vi "write acquisition config.vi"(8 "error in (no error)":errorcluster, 11 "Channel in":refnum<class "SPARC4_Channel.lvclass">) -> (0 "error out":errorcluster, 3 "Channel out":refnum<class "SPARC4_Channel.lvclass">)   [LabVIEW 2018, in "SPARC4_Channel.lvclass"]
uses:
  SPARC4_Channel.lvclass
  C:/Users/Denis/Desktop/S4ACS/S4ACS/Channel/Channel.lvclass
  SPARC4_Channel.lvclass/SPARC4_Channel.ctl
  Sim_CCD/Sim_CCD.lvclass
  Channel/Channel.lvclass
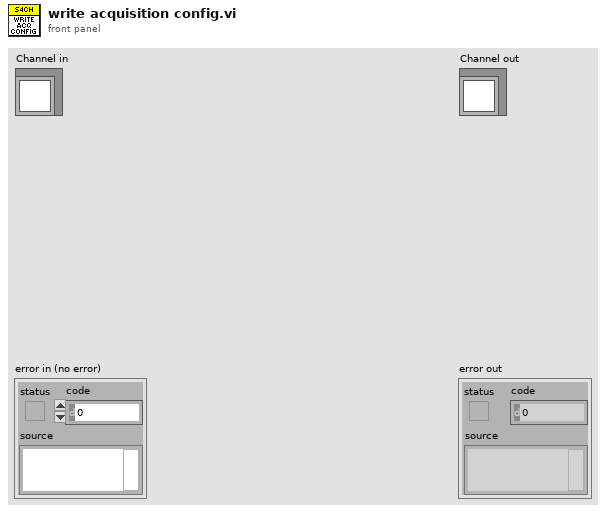
[diagram p1: front panel]
types:
  T1 = cluster{"#CYCLES":errorcluster, "SUFFIX":errorcluster}
  T2 = cluster{"#SEQS":errorcluster, "WAVEPLATE_POS":errorcluster}
  T3 = cluster{"State Machine.lvclass":refnum<class "State Machine.lvclass">, "RxTx.lvclass":refnum<class "RxTx.lvclass">, "Save_Header_RxTx.lvclass":refnum<class "RxTx.lvclass">, "Status SM.lvclass":refnum<class "State Machine.lvclass">, "Status RxTx.lvclass":refnum<class "RxTx.lvclass">, "servers array":refnum<class "Server.lvclass">[], "Events log file.lvclass":refnum<class "Log File.lvclass">, "Errors log file.lvclass":refnum<class "Log File.lvclass">, "Keywords log file.lvclass":refnum<class "Log File.lvclass">, "Sim_CCD.lvclass":refnum<class "Sim_CCD.lvclass">}
  T4 = cluster{"EXPTIME":errorcluster, "#FRAMES":errorcluster}
  T5 = cluster{"#SEQS":u32, "WAVEPLATE_POS":u16, "Waveplate positions":u8[]}
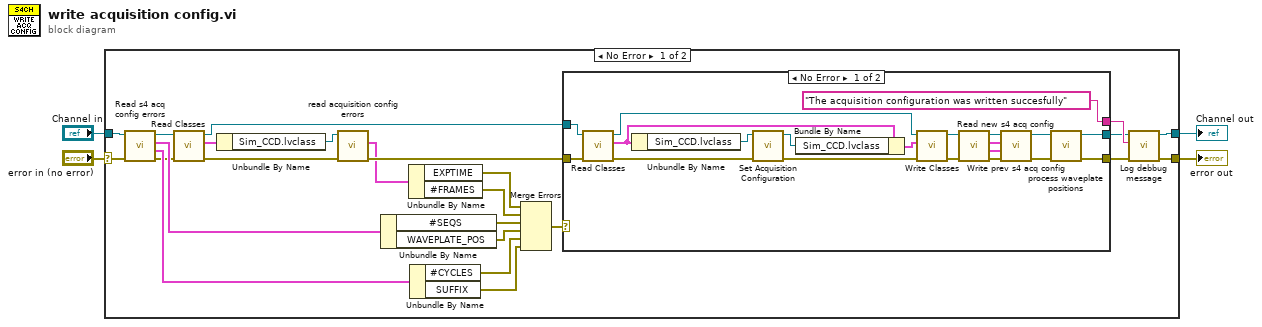
[diagram p0: block diagram]
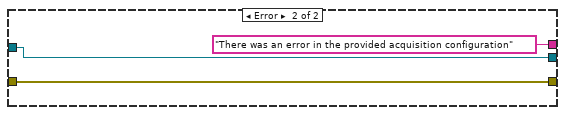
[diagram p2: hidden frame]
diagram:
  n1 = case shown="No Error" "error in (no error)" {
    selector: "error in (no error)" -> [w10 w53]
    tunnel: [w24 w53] -> w3
    tunnel: [w25 w52] -> w1
    tunnel: "Channel in" -> [w14 w52]
    frame No Error {
      n2 = call "Read s4 acq config errors.vi"("error in (no error)"=w10, "SPARC4_Channel in"=w14) -> ("error out"=w9:errorcluster, "acquisition config errors"=w19:T1, "s4 acq config errors"=w20:T2, "SPARC4_Channel out"=w13:refnum<class "SPARC4_Channel.lvclass">)  [unwired: 6 in]
      n3 = call-dynamic "Read Classes.vi"("error in (no error)"=w9, "Channel in"=w13) -> ("error out"=w8:errorcluster, "Classes"=w12:T3, "Channel out"=w7:refnum<class "SPARC4_Channel.lvclass">)  [unwired: 7 in]
      n4 = Unbundle By Name(w12) -> ("Sim_CCD.lvclass"=w11:refnum<class "Sim_CCD.lvclass">)
      n5 = call "read acquisition config errors.vi"("error in (no error)"=w8, "Simulated Camera in"=w11) -> ("error out"=w28:errorcluster, "acq config errors"=w27:T4)  [unwired: 7 in, 1 out]
      n6 = Unbundle By Name(w20) -> ("#SEQS"=w15:errorcluster, "WAVEPLATE_POS"=w16:errorcluster)
      n7 = Unbundle By Name(w27) -> ("EXPTIME"=w6:errorcluster, "#FRAMES"=w5:errorcluster)
      n8 = Unbundle By Name(w19) -> ("#CYCLES"=w17:errorcluster, "SUFFIX"=w18:errorcluster)
      n9 = Merge Errors(w6, w5, w15, w16, w17, w18) -> (w26:errorcluster)
      n10 = case shown="No Error" w26 {
        tunnel: w28 -> [w42 w51]
        tunnel: [w46 w51] -> w23
        tunnel: ["The acquisition configuration was written succesfully" ("String") "There was an error in the provided acquisition configuration" ("String")] -> w22
        tunnel: w7 -> [w45 w49]
        tunnel: [w47 w49] -> w21
        frame No Error {
          n11 = call-dynamic "Read Classes.vi"("error in (no error)"=w42, "Channel in"=w45) -> ("error out"=w43:errorcluster, "Classes"=w41:T3, "Channel out"=w39:refnum<class "SPARC4_Channel.lvclass">)  [unwired: 7 in]
          n12 = Unbundle By Name(w41) -> ("Sim_CCD.lvclass"=w44:refnum<class "Sim_CCD.lvclass">)
          n13 = call-dynamic "Set Acquisition Configuration.vi"("error in (no error)"=w43, "CCDCamera in"=w44) -> ("error out"=w37:errorcluster, "CCDCamera out"=w38:refnum<class "Sim_CCD.lvclass">)  [unwired: 8 in]
          n14 = Bundle By Name(cluster=w41, "Sim_CCD.lvclass"=w38) -> (w40:T3)
          n15 = call-dynamic "Write Classes.vi"("error in (no error)"=w37, "Classes"=w40, "Channel in"=w39) -> ("error out"=w35:errorcluster, "Channel out"=w36:refnum<class "SPARC4_Channel.lvclass">)  [unwired: 7 in]
          n16 = call "Read new s4 acq config.vi"("error in (no error)"=w35, "SPARC4_Channel in"=w36) -> ("error out"=w34:errorcluster, "new acq config"=w31:cluster{"suffix":string, "#CYCLES":u32}, "new s4 acq config"=w32:T5, "SPARC4_Channel out"=w33:refnum<class "SPARC4_Channel.lvclass">)  [unwired: 6 in]
          n17 = call "Write prev s4 acq config.vi"("error in (no error)"=w34, "prev SET parameters"=w31, "prev s4 acq config"=w32, "SPARC4_Channel in"=w33) -> ("error out"=w29:errorcluster, "SPARC4_Channel out"=w30:refnum<class "SPARC4_Channel.lvclass">)  [unwired: 6 in]
          n18 = call "process waveplate positions.vi"("error in (no error)"=w29, "Channel in"=w30) -> ("error out"=w46:errorcluster, "Channel out"=w47:refnum<class "SPARC4_Channel.lvclass">)  [unwired: 8 in]
        }
        frame Error {
        }
      }
      n19 = call "Log debbug message.vi"("error in (no error)"=w23, "String"=w22, "Channel in"=w21) -> ("error out"=w24:errorcluster, "Channel out"=w25:refnum<class "SPARC4_Channel.lvclass">)  [unwired: 7 in]
    }
    frame Error {
    }
  }
  "error out" <- w3
  "Channel out" <- w1
